vi "Read Source.vi"(8 "Error In":errorcluster, 11 "Node In":refnum<class "Root.lvclass">) -> (0 "Error Out":errorcluster, 2 "Source":string, 3 "Node Out":refnum<class "Root.lvclass">)   [LabVIEW 2018, in "Toolkit.lvlib" / "Nodes.lvlib" / "Root.lvclass"]
uses:
  Root.lvclass
  NonTerminal/NonTerminal.lvclass
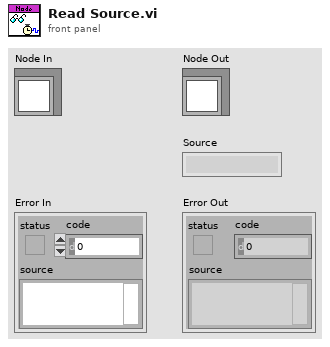
[diagram p1: front panel]
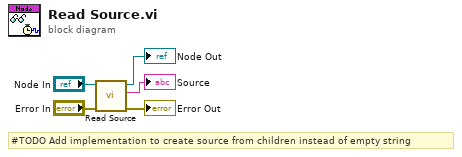
[diagram p0: block diagram]
diagram:
  # "#TODO Add implementation to create source from children instead of empty string"
  n1 = call-parent "Read Source.vi"("Error In"="Error In", "Node In"="Node In") -> ("Error Out"=→"Error Out":errorcluster, "Source"=→"Source":string, "Node Out"=→"Node Out":refnum<class "Root.lvclass">)  [unwired: 7 in]
